vi "main.vi"() -> ()   [LabVIEW 2023] (continued)
FF\tFF\tFF\tFF\tFF\tFF\r\n      2747  1FFFFFFF   00000004    8        00\t00\tFF\tFF\tFF\tFF\tFF\tFF\r\n      2746  18F121F0   00000004    8        09\t19\t00\t00\tFF\tFF\tB0\t01\r\n      2745  18F106A7   00000004    8        00\tF7\tFF\tFF\tFF\tFF\tFF\tA7\r\n      2745  0CF104A7   00000004    8        F0\t60\t22\tFC\tFF\tFF\tFF\t53\r\n      2744  0CF103A7   00000004    8        17\t1F\t08\t60\tB1\t1F\t08\t53\r\n      2783  0CF101A7   00000004    8        68\t00\t97\tCC\t00\t16\t39\tA5\r\n      2782  1FFFFFFF   00000004    8        00\t00\tFF\tFF\tFF\tFF\tFF\tFF\r\n      2772  1FFFFFFF   00000004    8        00\t00\tFF\tFF\tFF\tFF\tFF\tFF\r\n      2763  0CF102A7   00000004    8        30\t75\tE0\t2E\t80\tFF\tFF\tFD\r\n      2763  0CF101A7   00000004    8        68\t00\t97\tCC\t00\t16\t39\tA4\r\n      2762  1FFFFFFF   00000004    8        00\t00\tFF\tFF\tFF\tFF\tFF\tFF\r\n      2752  1FFFFFFF   00000004    8        00\t00\tFF\tFF\tFF\tFF\tFF\tFF\r\n      2747  1FFFFFFF   00000004    8        00\t00\tFF\tFF\tFF\tFF\tFF\tFF\r\n      2746  18F121F0   00000004    8        09\t19\t00\t00\tFF\tFF\tB0\t01\r\n      2745  18F106A7   00000004    8        00\tF7\tFF\tFF\tFF\tFF\tFF\tA7\r\n      2745  0CF104A7   00000004    8        F0\t60\t22\tFC\tFF\tFF\tFF\t53\r\n      2783  0CF102A7   00000004    8        30\t75\tE0\t2E\t80\tFF\tFF\tFD\r\n      2783  0CF101A7   00000004    8        68\t00\t97\tCC\t00\t16\t39\tA5\r\n      2782  1FFFFFFF   00000004    8        00\t00\tFF\tFF\tFF\tFF\tFF\tFF\r\n      2772  1FFFFFFF   00000004    8        00\t00\tFF\tFF\tFF\tFF\tFF\tFF\r\n      2763  0CF102A7   00000004    8        30\t75\tE0\t2E\t80\tFF\tFF\tFD\r\n      2763  0CF101A7   00000004    8        68\t00\t97\tCC\t00\t16\t39\tA4\r\n      2762  1FFFFFFF   00000004    8        00\t00\tFF\tFF\tFF\tFF\tFF\tFF\r\n      2752  1FFFFFFF   00000004    8        00\t00\tFF\tFF\tFF\tFF\tFF\tFF\r\n      2747  1FFFFFFF   00000004    8        00\t00\tFF\tFF\tFF\tFF\tFF\tFF\r\n      2746  18F121F0   00000004    8        09\t19\t00\t00\tFF\tFF\tB0\t01\r\n      2745  18F106A7   00000004    8        00\tF7\tFF\tFF\tFF\tFF\tFF\tA7\r\n      2792  1FFFFFFF   00000004    8        00\t00\tFF\tFF\tFF\tFF\tFF\tFF\r\n      2783  0CF102A7   00000004    8        30\t75\tE0\t2E\t80\tFF\tFF\tFD\r\n      2783  0CF101A7   00000004    8        68\t00\t97\tCC\t00\t16\t39\tA5\r\n      2782  1FFFFFFF   00000004    8        00\t00\tFF\tFF\tFF\tFF\tFF\tFF\r\n      2772  1FFFFFFF   00000004    8        00\t00\tFF\tFF\tFF\tFF\tFF\tFF\r\n      2763  0CF102A7   00000004    8        30\t75\tE0\t2E\t80\tFF\tFF\tFD\r\n      2763  0CF101A7   00000004    8        68\t00\t97\tCC\t00\t16\t39\tA4\r\n      2762  1FFFFFFF   00000004    8        00\t00\tFF\tFF\tFF\tFF\tFF\tFF\r\n      2752  1FFFFFFF   00000004    8        00\t00\tFF\tFF\tFF\tFF\tFF\tFF\r\n      2747  1FFFFFFF   00000004    8        00\t00\tFF\tFF\tFF\tFF\tFF\tFF\r\n      2746  18F121F0   00000004    8        09\t19\t00\t00\tFF\tFF\tB0\t01\r\n      2793  18F106A7   00000004    8        00\tF7\tFF\tFF\tFF\tFF\tFF\tA8\r\n      2792  1FFFFFFF   00000004    8        00\t00\tFF\tFF\tFF\tFF\tFF\tFF\r\n      2783  0CF102A7   00000004    8        30\t75\tE0\t2E\t80\tFF\tFF\tFD\r\n      2783  0CF101A7   00000004    8        68\t00\t97\tCC\t00\t16\t39\tA5\r\n      2782  1FFFFFFF   00000004    8        00\t00\tFF\tFF\tFF\tFF\tFF\tFF\r\n      2772  1FFFFFFF   00000004    8        00\t00\tFF\tFF\tFF\tFF\tFF\tFF\r\n      2763  0CF102A7   00000004    8        30\t75\tE0\t2E\t80\tFF\tFF\tFD\r\n      2763  0CF101A7   00000004    8        68\t00\t97\tCC\t00\t16\t39\tA4\r\n      2762  1FFFFFFF   00000004    8        00\t00\tFF\tFF\tFF\tFF\tFF\tFF\r\n      2752  1FFFFFFF   00000004    8        00\t00\tFF\tFF\tFF\tFF\tFF\tFF\r\n      2747  1FFFFFFF   00000004    8        00\t00\tFF\tFF\tFF\tFF\tFF\tFF\r\n      2802  1FFFFFFF   00000004    8        00\t00\tFF\tFF\tFF\tFF\tFF\tFF\r\n      2793  18F106A7   00000004    8        00\tF7\tFF\tFF\tFF\tFF\tFF\tA8\r\n      2792  1FFFFFFF   00000004    8        00\t00\tFF\tFF\tFF\tFF\tFF\tFF\r\n      2783  0CF102A7   00000004    8        30\t75\tE0\t2E\t80\tFF\tFF\tFD\r\n      2783  0CF101A7   00000004    8        68\t00\t97\tCC\t00\t16\t39\tA5\r\n      2782  1FFFFFFF   00000004    8        00\t00\tFF\tFF\tFF\tFF\tFF\tFF\r\n      2772  1FFFFFFF   00000004    8        00\t00\tFF\tFF\tFF\tFF\tFF\tFF\r\n      2763  0CF102A7   00000004    8        30\t75\tE0\t2E\t80\tFF\tFF\tFD\r\n      2763  0CF101A7   00000004    8        68\t00\t97\tCC\t00\t16\t39\tA4\r\n      2762  1FFFFFFF   00000004    8        00\t00\tFF\tFF\tFF\tFF\tFF\tFF\r\n      2752  1FFFFFFF   00000004    8        00\t00\tFF\tFF\tFF\tFF\tFF\tFF\r\n      2803  0CF101A7   00000004    8        68\t00\t97\tCC\t00\t16\t39\tA6\r\n      2802  1FFFFFFF   00000004    8        00\t00\tFF\tFF\tFF\tFF\tFF\tFF\r\n      2793  18F106A7   00000004    8        00\tF7\tFF\tFF\tFF\tFF\tFF\tA8\r\n      2792  1FFFFFFF   00000004    8        00\t00\tFF\tFF\tFF\tFF\tFF\tFF\r\n      2783  0CF102A7   00000004    8        30\t75\tE0\t2E\t80\tFF\tFF\tFD\r\n      2783  0CF101A7   00000004    8        68\t00\t97\tCC\t00\t16\t39\tA5\r\n      2782  1FFFFFFF   00000004    8        00\t00\tFF\tFF\tFF\tFF\tFF\tFF\r\n      2772  1FFFFFFF   00000004    8        00\t00\tFF\tFF\tFF\tFF\tFF\tFF\r\n      2763  0CF102A7   00000004    8        30\t75\tE0\t2E\t80\tFF\tFF\tFD\r\n      2763  0CF101A7   00000004    8        68\t00\t97\tCC\t00\t16\t39\tA4\r\n      2762  1FFFFFFF   00000004    8        00\t00\tFF\tFF\tFF\tFF\tFF\tFF\r\n      2803  0CF102A7   00000004    8        30\t75\tE0\t2E\t80\tFF\tFF\tFD\r\n      2803  0CF101A7   00000004    8        68\t00\t97\tCC\t00\t16\t39\tA6\r\n      2802  1FFFFFFF   00000004    8        00\t00\tFF\tFF\tFF\tFF\tFF\tFF\r\n      2793  18F106A7   00000004    8        00\tF7\tFF\tFF\tFF\tFF\tFF\tA8\r\n      2792  1FFFFFFF   00000004    8        00\t00\tFF\tFF\tFF\tFF\tFF\tFF\r\n      2783  0CF102A7   00000004    8        30\t75\tE0\t2E\t80\tFF\tFF\tFD\r\n      2783  0CF101A7   00000004    8        68\t00\t97\tCC\t00\t16\t39\tA5\r\n      2782  1FFFFFFF   00000004    8        00\t00\tFF\tFF\tFF\tFF\tFF\tFF\r\n      2772  1FFFFFFF   00000004    8        00\t00\tFF\tFF\tFF\tFF\tFF\tFF\r\n      2763  0CF102A7   00000004    8        30\t75\tE0\t2E\t80\tFF\tFF\tFD\r\n      2763  0CF101A7   00000004    8        68\t00\t97\tCC\t00\t16\t39\tA4\r\n      2812  1FFFFFFF   00000004    8        00\t00\tFF\tFF\tFF\tFF\tFF\tFF\r\n      2803  0CF102A7   00000004    8        30\t75\tE0\t2E\t80\tFF\tFF\tFD\r\n      2803  0CF101A7   00000004    8        68\t00\t97\tCC\t00\t16\t39\tA6\r\n      2802  1FFFFFFF   00000004    8        00\t00\tFF\tFF\tFF\tFF\tFF\tFF\r\n      2793  18F106A7   00000004    8        00\tF7\tFF\tFF\tFF\tFF\tFF\tA8\r\n      2792  1FFFFFFF   00000004    8        00\t00\tFF\tFF\tFF\tFF\tFF\tFF\r\n      2783  0CF102A7   00000004    8        30\t75\tE0\t2E\t80\tFF\tFF\tFD\r\n      2783  0CF101A7   00000004    8        68\t00\t97\tCC\t00\t16\t39\tA5\r\n      2782  1FFFFFFF   00000004    8        00\t00\tFF\tFF\tFF\tFF\tFF\tFF\r\n      2772  1FFFFFFF   00000004    8        00\t00\tFF\tFF\tFF\tFF\tFF\tFF\r\n      2763  0CF102A7   00000004    8        30\t75\tE0\t2E\t80\tFF\tFF\tFD\r\n      2822  1FFFFFFF   00000004    8        00\t00\tFF\tFF\tFF\tFF\tFF\tFF\r\n      2812  1FFFFFFF   00000004    8        00\t00\tFF\tFF\tFF\tFF\tFF\tFF\r\n      2803  0CF102A7   00000004    8        30\t75\tE0\t2E\t80\tFF\tFF\tFD\r\n      2803  0CF101A7   00000004    8        68\t00\t97\tCC\t00\t16\t39\tA6\r\n      2802  1FFFFFFF   00000004    8        00\t00\tFF\tFF\tFF\tFF\tFF\tFF\r\n      2793  18F106A7   00000004    8        00\tF7\tFF\tFF\tFF\tFF\tFF\tA8\r\n      2792  1FFFFFFF   00000004    8        00\t00\tFF\tFF\tFF\tFF\tFF\tFF\r\n      2783  0CF102A7   00000004    8        30\t75\tE0\t2E\t80\tFF\tFF\tFD\r\n      2783  0CF101A7   00000004    8        68\t00\t97\tCC\t00\t16\t39\tA5\r\n      2782  1FFFFFFF   00000004    8        00\t00\tFF\tFF\tFF\tFF\tFF\tFF\r\n      2772  1FFFFFFF   00000004    8        00\t00\tFF\tFF\tFF\tFF\tFF\tFF\r\n      2823  0CF101A7   00000004    8        68\t00\t97\tCC\t00\t16\t39\tA7\r\n      2822  1FFFFFFF   00000004    8        00\t00\tFF\tFF\tFF\tFF\tFF\tFF\r\n      2812  1FFFFFFF   00000004    8        00\t00\tFF\tFF\tFF\tFF\tFF\tFF\r\n      2803  0CF102A7   00000004    8        30\t75\tE0\t2E\t80\tFF\tFF\tFD\r\n      2803  0CF101A7   00000004    8        68\t00\t97\tCC\t00\t16\t39\tA6\r\n      2802  1FFFFFFF   00000004    8        00\t00\tFF\tFF\tFF\tFF\tFF\tFF\r\n      2793  18F106A7   00000004    8        00\tF7\tFF\tFF\tFF\tFF\tFF\tA8\r\n      2792  1FFFFFFF   00000004    8        00\t00\tFF\tFF\tFF\tFF\tFF\tFF\r\n      2783  0CF102A7   00000004    8        30\t75\tE0\t2E\t80\tFF\tFF\tFD\r\n      2783  0CF101A7   00000004    8        68\t00\t97\tCC\t00\t16\t39\tA5\r\n      2782  1FFFFFFF   00000004    8        00\t00\tFF\tFF\tFF\tFF\tFF\tFF\r\n      2823  0CF102A7   00000004    8        30\t75\tE0\t2E\t80\tFF\tFF\tFD\r\n      2823  0CF101A7   00000004    8        68\t00\t97\tCC\t00\t16\t39\tA7\r\n      2822  1FFFFFFF   00000004    8        00\t00\tFF\tFF\tFF\tFF\tFF\tFF\r\n      2812  1FFFFFFF   00000004    8        00\t00\tFF\tFF\tFF\tFF\tFF\tFF\r\n      2803  0CF102A7   00000004    8        30\t75\tE0\t2E\t80\tFF\tFF\tFD\r\n      2803  0CF101A7   00000004    8        68\t00\t97\tCC\t00\t16\t39\tA6\r\n      2802  1FFFFFFF   00000004    8        00\t00\tFF\tFF\tFF\tFF\tFF\tFF\r\n      2793  18F106A7   00000004    8        00\tF7\tFF\tFF\tFF\tFF\tFF\tA8\r\n      2792  1FFFFFFF   00000004    8        00\t00\tFF\tFF\tFF\tFF\tFF\tFF\r\n      2783  0CF102A7   00000004    8        30\t75\tE0\t2E\t80\tFF\tFF\tFD\r\n      2783  0CF101A7   00000004    8        68\t00\t97\tCC\t00\t16\t39\tA5\r\n      2832  1FFFFFFF   00000004    8        00\t00\tFF\tFF\tFF\tFF\tFF\tFF\r\n      2823  0CF102A7   00000004    8        30\t75\tE0\t2E\t80\tFF\tFF\tFD\r\n      2823  0CF101A7   00000004    8        68\t00\t97\tCC\t00\t16\t39\tA7\r\n      2822  1FFFFFFF   00000004    8        00\t00\tFF\tFF\tFF\tFF\tFF\tFF\r\n      2812  1FFFFFFF   00000004    8        00\t00\tFF\tFF\tFF\tFF\tFF\tFF\r\n      2803  0CF102A7   00000004    8        30\t75\tE0\t2E\t80\tFF\tFF\tFD\r\n      2803  0CF101A7   00000004    8        68\t00\t97\tCC\t00\t16\t39\tA6\r\n      2802  1FFFFFFF   00000004    8        00\t00\tFF\tFF\tFF\tFF\tFF\tFF\r\n      2793  18F106A7   00000004    8        00\tF7\tFF\tFF\tFF\tFF\tFF\tA8\r\n      2792  1FFFFFFF   00000004    8        00\t00\tFF\tFF\tFF\tFF\tFF\tFF\r\n      2783  0CF102A7   00000004    8        30\t75\tE0\t2E\t80\tFF\tFF\tFD\r\n      2841  18F11FF0   00000004    8        FF\t3F\t90\t68\t88\t1B\t10\t4C\r\n      2832  1FFFFFFF   00000004    8        00\t00\tFF\tFF\tFF\tFF\tFF\tFF\r\n      2823  0CF102A7   00000004    8        30\t75\tE0\t2E\t80\tFF\tFF\tFD\r\n      2823  0CF101A7   00000004    8        68\t00\t97\tCC\t00\t16\t39\tA7\r\n      2822  1FFFFFFF   00000004    8        00\t00\tFF\tFF\tFF\tFF\tFF\tFF\r\n      2812  1FFFFFFF   00000004    8        00\t00\tFF\tFF\tFF\tFF\tFF\tFF\r\n      2803  0CF102A7   00000004    8        30\t75\tE0\t2E\t80\tFF\tFF\tFD\r\n      2803  0CF101A7   00000004    8        68\t00\t97\tCC\t00\t16\t39\tA6\r\n      2802  1FFFFFFF   00000004    8        00\t00\tFF\tFF\tFF\tFF\tFF\tFF\r\n      2793  18F106A7   00000004    8        00\tF7\tFF\tFF\tFF\tFF\tFF\tA8\r\n      2792  1FFFFFFF   00000004    8        00\t00\tFF\tFF\tFF\tFF\tFF\tFF\r\n      2842  18F120F0   00000004    8        2B\t75\t60\tB1\tB0\t01\tFF\tFF\r\n      2841  18F11FF0   00000004    8        FF\t3F\t90\t68\t88\t1B\t10\t4C\r\n      2832  1FFFFFFF   00000004    8        00\t00\tFF\tFF\tFF\tFF\tFF\tFF\r\n      2823  0CF102A7   00000004    8        30\t75\tE0\t2E\t80\tFF\tFF\tFD\r\n      2823  0CF101A7   00000004    8        68\t00\t97\tCC\t00\t16\t39\tA7\r\n      2822  1FFFFFFF   00000004    8        00\t00\tFF\tFF\tFF\tFF\tFF\tFF\r\n      2812  1FFFFFFF   00000004    8        00\t00\tFF\tFF\tFF\tFF\tFF\tFF\r\n      2803  0CF102A7   00000004    8        30\t75\tE0\t2E\t80\tFF\tFF\tFD\r\n      2803  0CF101A7   00000004    8        68\t00\t97\tCC\t00\t16\t39\tA6\r\n      2802  1FFFFFFF   00000004    8        00\t00\tFF\tFF\tFF\tFF\tFF\tFF\r\n      2793  18F106A7   00000004    8        00\tF7\tFF\tFF\tFF\tFF\tFF\tA8\r\n      2843  0CF101A7   00000004    8        68\t00\t97\tCC\t00\t16\t39\tA8\r\n      2842  18F120F0   00000004    8        2B\t75\t60\tB1\tB0\t01\tFF\tFF\r\n      2841  18F11FF0   00000004    8        FF\t3F\t90\t68\t88\t1B\t10\t4C\r\n      2832  1FFFFFFF   00000004    8        00\t00\tFF\tFF\tFF\tFF\tFF\tFF\r\n      2823  0CF102A7   00000004    8        30\t75\tE0\t2E\t80\tFF\tFF\tFD\r\n      2823  0CF101A7   00000004    8        68\t00\t97\tCC\t00\t16\t39\tA7\r\n      2822  1FFFFFFF   00000004    8        00\t00\tFF\tFF\tFF\tFF\tFF\tFF\r\n      2812  1FFFFFFF   00000004    8        00\t00\tFF\tFF\tFF\tFF\tFF\tFF\r\n      2803  0CF102A7   00000004    8        30\t75\tE0\t2E\t80\tFF\tFF\tFD\r\n      2803  0CF101A7   00000004    8        68\t00\t97\tCC\t00\t16\t39\tA6\r\n      2802  1FFFFFFF   00000004    8        00\t00\tFF\tFF\tFF\tFF\tFF\tFF\r\n      2843  0C3C4D4A   00000004    8        BE\tFF\tFF\t7F\t18\tFF\tFF\t54\r\n      2843  0CF101A7   00000004    8        68\t00\t97\tCC\t00\t16\t39\tA8\r\n      2842  18F120F0   00000004    8        2B\t75\t60\tB1\tB0\t01\tFF\tFF\r\n      2841  18F11FF0   00000004    8        FF\t3F\t90\t68\t88\t1B\t10\t4C\r\n      2832  1FFFFFFF   00000004    8        00\t00\tFF\tFF\tFF\tFF\tFF\tFF\r\n      2823  0CF102A7   00000004    8        30\t75\tE0\t2E\t80\tFF\tFF\tFD\r\n      2823  0CF101A7   00000004    8        68\t00\t97\tCC\t00\t16\t39\tA7\r\n      2822  1FFFFFFF   00000004    8        00\t00\tFF\tFF\tFF\tFF\tFF\tFF\r\n      2812  1FFFFFFF   00000004    8        00\t00\tFF\tFF\tFF\tFF\tFF\tFF\r\n      2803  0CF102A7   00000004    8        30\t75\tE0\t2E\t80\tFF\tFF\tFD\r\n      2803  0CF101A7   00000004    8        68\t00\t97\tCC\t00\t16\t39\tA6\r\n      2844  0CF102A7   00000004    8        30\t75\tE0\t2E\t80\tFF\tFF\tFD\r\n      2843  0C3C4D4A   00000004    8        BE\tFF\tFF\t7F\t18\tFF\tFF\t54\r\n      2843  0CF101A7   00000004    8        68\t00\t97\tCC\t00\t16\t39\tA8\r\n      2842  18F120F0   00000004    8        2B\t75\t60\tB1\tB0\t01\tFF\tFF\r\n      2841  18F11FF0   00000004    8        FF\t3F\t90\t68\t88\t1B\t10\t4C\r\n      2832  1FFFFFFF   00000004    8        00\t00\tFF\tFF\tFF\tFF\tFF\tFF\r\n      2823  0CF102A7   00000004    8        30\t75\tE0\t2E\t80\tFF\tFF\tFD\r\n      2823  0CF101A7   00000004    8        68\t00\t97\tCC\t00\t16\t39\tA7\r\n      2822  1FFFFFFF   00000004    8        00\t00\tFF\tFF\tFF\tFF\tFF\tFF\r\n      2812  1FFFFFFF   00000004    8        00\t00\tFF\tFF\tFF\tFF\tFF\tFF\r\n      2803  0CF102A7   00000004    8        30\t75\tE0\t2E\t80\tFF\tFF\tFD\r\n      2844  0CF103A7   00000004    8        17\t1F\t08\t60\tB1\t1F\t08\t54\r\n      2844  0CF102A7   00000004    8        30\t75\tE0\t2E\t80\tFF\tFF\tFD\r\n      2843  0C3C4D4A   00000004    8        BE\tFF\tFF\t7F\t18\tFF\tFF\t54\r\n      2843  0CF101A7   00000004    8        68\t00\t97\tCC\t00\t16\t39\tA8\r\n      2842  18F120F0   00000004    8        2B\t75\t60\tB1\tB0\t01\tFF\tFF\r\n      2841  18F11FF0   00000004    8        FF\t3F\t90\t68\t88\t1B\t10\t4C\r\n      2832  1FFFFFFF   00000004    8        00\t00\tFF\tFF\tFF\tFF\tFF\tFF\r\n      2823  0CF102A7   00000004    8        30\t75\tE0\t2E\t80\tFF\tFF\tFD\r\n      2823  0CF101A7   00000004    8        68\t00\t97\tCC\t00\t16\t39\tA7\r\n      2822  1FFFFFFF   00000004    8        00\t00\tFF\tFF\tFF\tFF\tFF\tFF\r\n      2812  1FFFFFFF   00000004    8        00\t00\tFF\tFF\tFF\tFF\tFF\tFF\r\n      2845  0CF104A7   00000004    8        F0\t60\t22\tFC\tFF\tFF\tFF\t54\r\n      2844  0CF103A7   00000004    8        17\t1F\t08\t60\tB1\t1F\t08\t54\r\n      2844  0CF102A7   00000004    8        30\t75\tE0\t2E\t80\tFF\tFF\tFD\r\n      2843  0C3C4D4A   00000004    8        BE\tFF\tFF\t7F\t18\tFF\tFF\t54\r\n      2843  0CF101A7   00000004    8        68\t00\t97\tCC\t00\t16\t39\tA8\r\n      2842  18F120F0   00000004    8        2B\t75\t60\tB1\tB0\t01\tFF\tFF\r\n      2841  18F11FF0   00000004    8        FF\t3F\t90\t68\t88\t1B\t10\t4C\r\n      2832  1FFFFFFF   00000004    8        00\t00\tFF\tFF\tFF\tFF\tFF\tFF\r\n      2823  0CF102A7   00000004    8        30\t75\tE0\t2E\t80\tFF\tFF\tFD\r\n      2823  0CF101A7   00000004    8        68\t00\t97\tCC\t00\t16\t39\tA7\r\n      2822  1FFFFFFF   00000004    8        00\t00\tFF\tFF\tFF\tFF\tFF\tFF\r\n      2845  18F106A7   00000004    8        00\tF7\tFF\tFF\tFF\tFF\tFF\tA9\r\n      2845  0CF104A7   00000004    8        F0\t60\t22\tFC\tFF\tFF\tFF\t54\r\n      2844  0CF103A7   00000004    8        17\t1F\t08\t60\tB1\t1F\t08\t54\r\n      2844  0CF102A7   00000004    8        30\t75\tE0\t2E\t80\tFF\tFF\tFD\r\n      2843  0C3C4D4A   00000004    8        BE\tFF\tFF\t7F\t18\tFF\tFF\t54\r\n      2843  0CF101A7   00000004    8        68\t00\t97\tCC\t00\t16\t39\tA8\r\n      2842  18F120F0   00000004    8        2B\t75\t60\tB1\tB0\t01\tFF\tFF\r\n      2841  18F11FF0   00000004    8        FF\t3F\t90\t68\t88\t1B\t10\t4C\r\n      2832  1FFFFFFF   00000004    8        00\t00\tFF\tFF\tFF\tFF\tFF\tFF\r\n      2823  0CF102A7   00000004    8        30\t75\tE0\t2E\t80\tFF\tFF\tFD\r\n      2823  0CF101A7   00000004    8        68\t00\t97\tCC\t00\t16\t39\tA7\r\n      2846  18F121F0   00000004    8        09\t19\t00\t00\tFF\tFF\tB0\t01\r\n      2845  18F106A7   00000004    8        00\tF7\tFF\tFF\tFF\tFF\tFF\tA9\r\n      2845  0CF104A7   00000004    8        F0\t60\t22\tFC\tFF\tFF\tFF\t54\r\n      2844  0CF103A7   00000004    8        17\t1F\t08\t60\tB1\t1F\t08\t54\r\n      2844  0CF102A7   00000004    8        30\t75\tE0\t2E\t80\tFF\tFF\tFD\r\n      2843  0C3C4D4A   00000004    8        BE\tFF\tFF\t7F\t18\tFF\tFF\t54\r\n      2843  0CF101A7   00000004    8        68\t00\t97\tCC\t00\t16\t39\tA8\r\n      2842  18F120F0   00000004    8        2B\t75\t60\tB1\tB0\t01\tFF\tFF\r\n      2841  18F11FF0   00000004    8        FF\t3F\t90\t68\t88\t1B\t10\t4C\r\n      2832  1FFFFFFF   00000004    8        00\t00\tFF\tFF\tFF\tFF\tFF\tFF\r\n      2823  0CF102A7   00000004    8        30\t75\tE0\t2E\t80\tFF\tFF\tFD\r\n      2847  1FFFFFFF   00000004    8        00\t00\tFF\tFF\tFF\tFF\tFF\tFF\r\n      2846  18F121F0   00000004    8        09\t19\t00\t00\tFF\tFF\tB0\t01\r\n      2845  18F106A7   00000004    8        00\tF7\tFF\tFF\tFF\tFF\tFF\tA9\r\n      2845  0CF104A7   00000004    8        F0\t60\t22\tFC\tFF\tFF\tFF\t54\r\n      2844  0CF103A7   00000004    8        17\t1F\t08\t60\tB1\t1F\t08\t54\r\n      2844  0CF102A7   00000004    8        30\t75\tE0\t2E\t80\tFF\tFF\tFD\r\n      2843  0C3C4D4A   00000004    8        BE\tFF\tFF\t7F\t18\tFF\tFF\t54\r\n      2843  0CF101A7   00000004    8        68\t00\t97\tCC\t00\t16\t39\tA8\r\n      2842  18F120F0   00000004    8        2B\t75\t60\tB1\tB0\t01\tFF\tFF\r\n      2841  18F11FF0   00000004    8        FF\t3F\t90\t68\t88\t1B\t10\t4C\r\n      2832  1FFFFFFF   00000004    8        00\t00\tFF\tFF\tFF\tFF\tFF\tFF\r\n      2852  1FFFFFFF   00000004    8        00\t20\tFF\tFF\tFF\tFF\tFF\tFF\r\n      2847  1FFFFFFF   00000004    8        00\t00\tFF\tFF\tFF\tFF\tFF\tFF\r\n      2846  18F121F0   00000004    8        09\t19\t00\t00\tFF\tFF\tB0\t01\r\n      2845  18F106A7   00000004    8        00\tF7\tFF\tFF\tFF\tFF\tFF\tA9\r\n      2845  0CF104A7   00000004    8        F0\t60\t22\tFC\tFF\tFF\tFF\t54\r\n      2844  0CF103A7   00000004    8        17\t1F\t08\t60\tB1\t1F\t08\t54\r\n      2844  0CF102A7   00000004    8        30\t75\tE0\t2E\t80\tFF\tFF\tFD\r\n      2843  0C3C4D4A   00000004    8        BE\tFF\tFF\t7F\t18\tFF\tFF\t54\r\n      2843  0CF101A7   00000004    8        68\t00\t97\tCC\t00\t16\t39\tA8\r\n      2842  18F120F0   00000004    8        2B\t75\t60\tB1\tB0\t01\tFF\tFF\r\n      2841  18F11FF0   00000004    8        FF\t3F\t90\t68\t88\t1B\t10\t4C\r\n      2862  1FFFFFFF   00000004    8        00\t20\tFF\tFF\tFF\tFF\tFF\tFF\r\n      2852  1FFFFFFF   00000004    8        00\t20\tFF\tFF\tFF\tFF\tFF\tFF\r\n      2847  1FFFFFFF   00000004    8        00\t00\tFF\tFF\tFF\tFF\tFF\tFF\r\n      2846  18F121F0   00000004    8        09\t19\t00\t00\tFF\tFF\tB0\t01\r\n      2845  18F106A7   00000004    8        00\tF7\tFF\tFF\tFF\tFF\tFF\tA9\r\n      2845  0CF104A7   00000004    8        F0\t60\t22\tFC\tFF\tFF\tFF\t54\r\n      2844  0CF103A7   00000004    8        17\t1F\t08\t60\tB1\t1F\t08\t54\r\n      2844  0CF102A7   00000004    8        30\t75\tE0\t2E\t80\tFF\tFF\tFD\r\n      2843  0C3C4D4A   00000004    8        BE\tFF\tFF\t7F\t18\tFF\tFF\t54\r\n      2843  0CF101A7   00000004    8        68\t00\t97\tCC\t00\t16\t39\tA8\r\n      2842  18F120F0   00000004    8        2B\t75\t60\tB1\tB0\t01\tFF\tFF\r\n      2863  0CF101A7   00000004    8        68\t00\t97\tCC\t00\t16\t39\tA9\r\n      2862  1FFFFFFF   00000004    8        00\t20\tFF\tFF\tFF\tFF\tFF\tFF\r\n      2852  1FFFFFFF   00000004    8        00\t20\tFF\tFF\tFF\tFF\tFF\tFF\r\n      2847  1FFFFFFF   00000004    8        00\t00\tFF\tFF\tFF\tFF\tFF\tFF\r\n      2846  18F121F0   00000004    8        09\t19\t00\t00\tFF\tFF\tB0\t01\r\n      2845  18F106A7   00000004    8        00\tF7\tFF\tFF\tFF\tFF\tFF\tA9\r\n      2845  0CF104A7   00000004    8        F0\t60\t22\tFC\tFF\tFF\tFF\t54\r\n      2844  0CF103A7   00000004    8        17\t1F\t08\t60\tB1\t1F\t08\t54\r\n      2844  0CF102A7   00000004    8        30\t75\tE0\t2E\t80\tFF\tFF\tFD\r\n      2843  0C3C4D4A   00000004    8        BE\tFF\tFF\t7F\t18\tFF\tFF\t54\r\n      2843  0CF101A7   00000004    8        68\t00\t97\tCC\t00\t16\t39\tA8\r\n      2863  0CF102A7   00000004    8        30\t75\tE0\t2E\t80\tFF\tFF\tFD\r\n      2863  0CF101A7   00000004    8        68\t00\t97\tCC\t00\t16\t39\tA9\r\n      2862  1FFFFFFF   00000004    8        00\t20\tFF\tFF\tFF\tFF\tFF\tFF\r\n      2852  1FFFFFFF   00000004    8        00\t20\tFF\tFF\tFF\tFF\tFF\tFF\r\n      2847  1FFFFFFF   00000004    8        00\t00\tFF\tFF\tFF\tFF\tFF\tFF\r\n      2846  18F121F0   00000004    8        09\t19\t00\t00\tFF\tFF\tB0\t01\r\n      2845  18F106A7   00000004    8        00\tF7\tFF\tFF\tFF\tFF\tFF\tA9\r\n      2845  0CF104A7   00000004    8        F0\t60\t22\tFC\tFF\tFF\tFF\t54\r\n      2844  0CF103A7   00000004    8        17\t1F\t08\t60\tB1\t1F\t08\t54\r\n      2844  0CF102A7   00000004    8        30\t75\tE0\t2E\t80\tFF\tFF\tFD\r\n      2843  0C3C4D4A   00000004    8        BE\tFF\tFF\t7F\t18\tFF\tFF\t54\r\n      2872  1FFFFFFF   00000004    8        00\t00\tFF\tFF\tFF\tFF\tFF\tFF\r\n      2863  0CF102A7   00000004    8        30\t75\tE0\t2E\t80\tFF\tFF\tFD\r\n      2863  0CF101A7   00000004    8        68\t00\t97\tCC\t00\t16\t39\tA9\r\n      2862  1FFFFFFF   00000004    8        00\t20\tFF\tFF\tFF\tFF\tFF\tFF\r\n      2852  1FFFFFFF   00000004    8        00\t20\tFF\tFF\tFF\tFF\tFF\tFF\r\n      2847  1FFFFFFF   00000004    8        00\t00\tFF\tFF\tFF\tFF\tFF\tFF\r\n      2846  18F121F0   00000004    8        09\t19\t00\t00\tFF\tFF\tB0\t01\r\n      2845  18F106A7   00000004    8        00\tF7\tFF\tFF\tFF\tFF\tFF\tA9\r\n      2845  0CF104A7   00000004    8        F0\t60\t22\tFC\tFF\tFF\tFF\t54\r\n      2844  0CF103A7   00000004    8        17\t1F\t08\t60\tB1\t1F\t08\t54\r\n      2844  0CF102A7   00000004    8        30\t75\tE0\t2E\t80\tFF\tFF\tFD\r\n      2882  1FFFFFFF   00000004    8        00\t00\tFF\tFF\tFF\tFF\tFF\tFF\r\n      2872  1FFFFFFF   00000004    8        00\t00\tFF\tFF\tFF\tFF\tFF\tFF\r\n      2863  0CF102A7   00000004    8        30\t75\tE0\t2E\t80\tFF\tFF\tFD\r\n      2863  0CF101A7   00000004    8        68\t00\t97\tCC\t00\t16\t39\tA9\r\n      2862  1FFFFFFF   00000004    8        00\t20\tFF\tFF\tFF\tFF\tFF\tFF\r\n      2852  1FFFFFFF   00000004    8        00\t20\tFF\tFF\tFF\tFF\tFF\tFF\r\n      2847  1FFFFFFF   00000004    8        00\t00\tFF\tFF\tFF\tFF\tFF\tFF\r\n      2846  18F121F0   00000004    8        09\t19\t00\t00\tFF\tFF\tB0\t01\r\n      2845  18F106A7   00000004    8        00\tF7\tFF\tFF\tFF\tFF\tFF\tA9\r\n      2845  0CF104A7   00000004    8        F0\t60\t22\tFC\tFF\tFF\tFF\t54\r\n      2844  0CF103A7   00000004    8        17\t1F\t08\t60\tB1\t1F\t08\t54\r\n      2883  0CF101A7   00000004    8        68\t00\t97\tCC\t00\t16\t39\tAA\r\n      2882  1FFFFFFF   00000004    8        00\t00\tFF\tFF\tFF\tFF\tFF\tFF\r\n      2872  1FFFFFFF   00000004    8        00\t00\tFF\tFF\tFF\tFF\tFF\tFF\r\n      2863  0CF102A7   00000004    8        30\t75\tE0\t2E\t80\tFF\tFF\tFD\r\n      2863  0CF101A7   00000004    8        68\t00\t97\tCC\t00\t16\t39\tA9\r\n      2862  1FFFFFFF   00000004    8        00\t20\tFF\tFF\tFF\tFF\tFF\tFF\r\n      2852  1FFFFFFF   00000004    8        00\t20\tFF\tFF\tFF\tFF\tFF\tFF\r\n      2847  1FFFFFFF   00000004    8        00\t00\tFF\tFF\tFF\tFF\tFF\tFF\r\n      2846  18F121F0   00000004    8        09\t19\t00\t00\tFF\tFF\tB0\t01\r\n      2845  18F106A7   00000004    8        00\tF7\tFF\tFF\tFF\tFF\tFF\tA9\r\n      2845  0CF104A7   00000004    8        F0\t60\t22\tFC\tFF\tFF\tFF\t54\r\n      2883  0CF102A7   00000004    8        30\t75\tE0\t2E\t80\tFF\tFF\tFD\r\n      2883  0CF101A7   00000004    8        68\t00\t97\tCC\t00\t16\t39\tAA\r\n      2882  1FFFFFFF   00000004    8        00\t00\tFF\tFF\tFF\tFF\tFF\tFF\r\n      2872  1FFFFFFF   00000004    8        00\t00\tFF\tFF\tFF\tFF\tFF\tFF\r\n      2863  0CF102A7   00000004    8        30\t75\tE0\t2E\t80\tFF\tFF\tFD\r\n      2863  0CF101A7   00000004    8        68\t00\t97\tCC\t00\t16\t39\tA9\r\n      2862  1FFFFFFF   00000004    8        00\t20\tFF\tFF\tFF\tFF\tFF\tFF\r\n      2852  1FFFFFFF   00000004    8        00\t20\tFF\tFF\tFF\tFF\tFF\tFF\r\n      2847  1FFFFFFF   00000004    8        00\t00\tFF\tFF\tFF\tFF\tFF\tFF\r\n      2846  18F121F0   00000004    8        09\t19\t00\t00\tFF\tFF\tB0\t01\r\n      2845  18F106A7   00000004    8        00\tF7\tFF\tFF\tFF\tFF\tFF\tA9\r\n      2892  1FFFFFFF   00000004    8        00\t20\tFF\tFF\tFF\tFF\tFF\tFF\r\n      2883  0CF102A7   00000004    8        30\t75\tE0\t2E\t80\tFF\tFF\tFD\r\n      2883  0CF101A7   00000004    8        68\t00\t97\tCC\t00\t16\t39\tAA\r\n      2882  1FFFFFFF   00000004    8        00\t00\tFF\tFF\tFF\tFF\tFF\tFF\r\n      2872  1FFFFFFF   00000004    8        00\t00\tFF\tFF\tFF\tFF\tFF\tFF\r\n      2863  0CF102A7   00000004    8        30\t75\tE0\t2E\t80\tFF\tFF\tFD\r\n      2863  0CF101A7   00000004    8        68\t00\t97\tCC\t00\t16\t39\tA9\r\n      2862  1FFFFFFF   00000004    8        00\t20\tFF\tFF\tFF\tFF\tFF\tFF\r\n      2852  1FFFFFFF   00000004    8        00\t20\tFF\tFF\tFF\tFF\tFF\tFF\r\n      2847  1FFFFFFF   00000004    8        00\t00\tFF\tFF\tFF\tFF\tFF\tFF\r\n      2846  18F121F0   00000004    8        09\t19\t00\t00\tFF\tFF\tB0\t01\r\n      2893  18F106A7   00000004    8        00\tF7\tFF\tFF\tFF\tFF\tFF\tAA\r\n      2892  1FFFFFFF   00000004    8        00\t20\tFF\tFF\tFF\tFF\tFF\tFF\r\n      2883  0CF102A7   00000004    8        30\t75\tE0\t2E\t80\tFF\tFF\tFD\r\n      2883  0CF101A7   00000004    8        68\t00\t97\tCC\t00\t16\t39\tAA\r\n      2882  1FFFFFFF   00000004    8        00\t00\tFF\tFF\tFF\tFF\tFF\tFF\r\n      2872  1FFFFFFF   00000004    8        00\t00\tFF\tFF\tFF\tFF\tFF\tFF\r\n      2863  0CF102A7   00000004    8        30\t75\tE0\t2E\t80\tFF\tFF\tFD\r\n      2863  0CF101A7   00000004    8        68\t00\t97\tCC\t00\t16\t39\tA9\r\n      2862  1FFFFFFF   00000004    8        00\t20\tFF\tFF\tFF\tFF\tFF\tFF\r\n      2852  1FFFFFFF   00000004    8        00\t20\tFF\tFF\tFF\tFF\tFF\tFF\r\n      2847  1FFFFFFF   00000004    8        00\t00\tFF\tFF\tFF\tFF\tFF\tFF\r\n      2902  1FFFFFFF   00000004    8        00\t20\tFF\tFF\tFF\tFF\tFF\tFF\r\n      2893  18F106A7   00000004    8        00\tF7\tFF\tFF\tFF\tFF\tFF\tAA\r\n      2892  1FFFFFFF   00000004    8        00\t20\tFF\tFF\tFF\tFF\tFF\tFF\r\n      2883  0CF102A7   00000004    8        30\t75\tE0\t2E\t80\tFF\tFF\tFD\r\n      2883  0CF101A7   00000004    8        68\t00\t97\tCC\t00\t16\t39\tAA\r\n      2882  1FFFFFFF   00000004    8        00\t00\tFF\tFF\tFF\tFF\tFF\tFF\r\n      2872  1FFFFFFF   00000004    8        00\t00\tFF\tFF\tFF\tFF\tFF\tFF\r\n      2863  0CF102A7   00000004    8        30\t75\tE0\t2E\t80\tFF\tFF\tFD\r\n      2863  0CF101A7   00000004    8        68\t00\t97\tCC\t00\t16\t39\tA9\r\n      2862  1FFFFFFF   00000004    8        00\t20\tFF\tFF\tFF\tFF\tFF\tFF\r\n      2852  1FFFFFFF   00000004    8        00\t20\tFF\tFF\tFF\tFF\tFF\tFF\r\n      2903  0CF101A7   00000004    8        68\t00\t97\tCC\t00\t16\t39\tAB\r\n      2902  1FFFFFFF   00000004    8        00\t20\tFF\tFF\tFF\tFF\tFF\tFF\r\n      2893  18F106A7   00000004    8        00\tF7\tFF\tFF\tFF\tFF\tFF\tAA\r\n      2892  1FFFFFFF   00000004    8        00\t20\tFF\tFF\tFF\tFF\tFF\tFF\r\n      2883  0CF102A7   00000004    8        30\t75\tE0\t2E\t80\tFF\tFF\tFD\r\n      2883  0CF101A7   00000004    8        68\t00\t97\tCC\t00\t16\t39\tAA\r\n      2882  1FFFFFFF   00000004    8        00\t00\tFF\tFF\tFF\tFF\tFF\tFF\r\n      2872  1FFFFFFF   00000004    8        00\t00\tFF\tFF\tFF\tFF\tFF\tFF\r\n      2863  0CF102A7   00000004    8        30\t75\tE0\t2E\t80\tFF\tFF\tFD\r\n      2863  0CF101A7   00000004    8        68\t00\t97\tCC\t00\t16\t39\tA9\r\n      2862  1FFFFFFF   00000004    8        00\t20\tFF\tFF\tFF\tFF\tFF\tFF\r\n      2903  0CF102A7   00000004    8        30\t75\tE0\t2E\t80\tFF\tFF\tFD\r\n      2903  0CF101A7   00000004    8        68\t00\t97\tCC\t00\t16\t39\tAB\r\n      2902  1FFFFFFF   00000004    8        00\t20\tFF\tFF\tFF\tFF\tFF\tFF\r\n      2893  18F106A7   00000004    8        00\tF7\tFF\tFF\tFF\tFF\tFF\tAA\r\n      2892  1FFFFFFF   00000004    8        00\t20\tFF\tFF\tFF\tFF\tFF\tFF\r\n      2883  0CF102A7   00000004    8        30\t75\tE0\t2E\t80\tFF\tFF\tFD\r\n      2883  0CF101A7   00000004    8        68\t00\t97\tCC\t00\t16\t39\tAA\r\n      2882  1FFFFFFF   00000004    8        00\t00\tFF\tFF\tFF\tFF\tFF\tFF\r\n      2872  1FFFFFFF   00000004    8        00\t00\tFF\tFF\tFF\tFF\tFF\tFF\r\n      2863  0CF102A7   00000004    8        30\t75\tE0\t2E\t80\tFF\tFF\tFD\r\n      2863  0CF101A7   00000004    8        68\t00\t97\tCC\t00\t16\t39\tA9\r\n      2912  1FFFFFFF   00000004    8        00\t20\tFF\tFF\tFF\tFF\tFF\tFF\r\n      2903  0CF102A7   00000004    8        30\t75\tE0\t2E\t80\tFF\tFF\tFD\r\n      2903  0CF101A7   00000004    8        68\t00\t97\tCC\t00\t16\t39\tAB\r\n      2902  1FFFFFFF   00000004    8        00\t20\tFF\tFF\tFF\tFF\tFF\tFF\r\n      2893  18F106A7   00000004    8        00\tF7\tFF\tFF\tFF\tFF\tFF\tAA\r\n      2892  1FFFFFFF   00000004    8        00\t20\tFF\tFF\tFF\tFF\tFF\tFF\r\n      2883  0CF102A7   00000004    8        30\t75\tE0\t2E\t80\tFF\tFF\tFD\r\n      2883  0CF101A7   00000004    8        68\t00\t97\tCC\t00\t16\t39\tAA\r\n      2882  1FFFFFFF   00000004    8        00\t00\tFF\tFF\tFF\tFF\tFF\tFF\r\n      2872  1FFFFFFF   00000004    8        00\t00\tFF\tFF\tFF\tFF\tFF\tFF\r\n      2863  0CF102A7   00000004    8        30\t75\tE0\t2E\t80\tFF\tFF\tFD\r\n      2922  1FFFFFFF   00000004    8        00\t20\tFF\tFF\tFF\tFF\tFF\tFF\r\n      2912  1FFFFFFF   00000004    8        00\t20\tFF\tFF\tFF\tFF\tFF\tFF\r\n      2903  0CF102A7   00000004    8        30\t75\tE0\t2E\t80\tFF\tFF\tFD\r\n      2903  0CF101A7   00000004    8        68\t00\t97\tCC\t00\t16\t39\tAB\r\n      2902  1FFFFFFF   00000004    8        00\t20\tFF\tFF\tFF\tFF\tFF\tFF\r\n      2893  18F106A7   00000004    8        00\tF7\tFF\tFF\tFF\tFF\tFF\tAA\r\n      2892  1FFFFFFF   00000004    8        00\t20\tFF\tFF\tFF\tFF\tFF\tFF\r\n      2883  0CF102A7   00000004    8        30\t75\tE0\t2E\t80\tFF\tFF\tFD\r\n      2883  0CF101A7   00000004    8        68\t00\t97\tCC\t00\t16\t39\tAA\r\n      2882  1FFFFFFF   00000004    8        00\t00\tFF\tFF\tFF\tFF\tFF\tFF\r\n      2872  1FFFFFFF   00000004    8        00\t00\tFF\tFF\tFF\tFF\tFF\tFF\r\n      2923  0CF101A7   00000004    8        68\t00\t97\tCC\t00\t16\t39\tAC\r\n      2922  1FFFFFFF   00000004    8        00\t20\tFF\tFF\tFF\tFF\tFF\tFF\r\n      2912  1FFFFFFF   00000004    8        00\t20\tFF\tFF\tFF\tFF\tFF\tFF\r\n      2903  0CF102A7   00000004    8        30\t75\tE0\t2E\t80\tFF\tFF\tFD\r\n      2903  0CF101A7   00000004    8        68\t00\t97\tCC\t00\t16\t39\tAB\r\n      2902  1FFFFFFF   00000004    8        00\t20\tFF\tFF\tFF\tFF\tFF\tFF\r\n      2893  18F106A7   00000004    8        00\tF7\tFF\tFF\tFF\tFF\tFF\tAA\r\n      2892  1FFFFFFF   00000004    8        00\t20\tFF\tFF\tFF\tFF\tFF\tFF\r\n      2883  0CF102A7   00000004    8        30\t75\tE0\t2E\t80\tFF\tFF\tFD\r\n      2883  0CF101A7   00000004    8        68\t00\t97\tCC\t00\t16\t39\tAA\r\n      2882  1FFFFFFF   00000004    8        00\t00\tFF\tFF\tFF\tFF\tFF\tFF\r\n      2923  0CF102A7   00000004    8        30\t75\tE0\t2E\t80\tFF\tFF\tFD\r\n      2923  0CF101A7   00000004    8        68\t00\t97\tCC\t00\t16\t39\tAC\r\n      2922  1FFFFFFF   00000004    8        00\t20\tFF\tFF\tFF\tFF\tFF\tFF\r\n      2912  1FFFFFFF   00000004    8        00\t20\tFF\tFF\tFF\tFF\tFF\tFF\r\n      2903  0CF102A7   00000004    8        30\t75\tE0\t2E\t80\tFF\tFF\tFD\r\n      2903  0CF101A7   00000004    8        68\t00\t97\tCC\t00\t16\t39\tAB\r\n      2902  1FFFFFFF   00000004    8        00\t20\tFF\tFF\tFF\tFF\tFF\tFF\r\n      2893  18F106A7   00000004    8        00\tF7\tFF\tFF\tFF\tFF\tFF\tAA\r\n      2892  1FFFFFFF   00000004    8        00\t20\tFF\tFF\tFF\tFF\tFF\tFF\r\n      2883  0CF102A7   00000004    8        30\t75\tE0\t2E\t80\tFF\tFF\tFD\r\n      2883  0CF101A7   00000004    8        68\t00\t97\tCC\t00\t16\t39\tAA\r\n      2932  1FFFFFFF   00000004    8        00\t00\tFF\tFF\tFF\tFF\tFF\tFF\r\n      2923  0CF102A7   00000004    8        30\t75\tE0\t2E\t80\tFF\tFF\tFD\r\n      2923  0CF101A7   00000004    8        68\t00\t97\tCC\t00\t16\t39\tAC\r\n      2922  1FFFFFFF   00000004    8        00\t20\tFF\tFF\tFF\tFF\tFF\tFF\r\n      2912  1FFFFFFF   00000004    8        00\t20\tFF\tFF\tFF\tFF\tFF\tFF\r\n      2903  0CF102A7   00000004    8        30\t75\tE0\t2E\t80\tFF\tFF\tFD\r\n      2903  0CF101A7   00000004    8        68\t00\t97\tCC\t00\t16\t39\tAB\r\n      2902  1FFFFFFF   00000004    8        00\t20\tFF\tFF\tFF\tFF\tFF\tFF\r\n      2893  18F106A7   00000004    8        00\tF7\tFF\tFF\tFF\tFF\tFF\tAA\r\n      2892  1FFFFFFF   00000004    8        00\t20\tFF\tFF\tFF\tFF\tFF\tFF\r\n      2883  0CF102A7   00000004    8        30\t75\tE0\t2E\t80\tFF\tFF\tFD\r\n      2941  18F11FF0   00000004    8        FF\t3F\t90\t68\t88\t1B\t10\t5C\r\n      2932  1FFFFFFF   00000004    8        00\t00\tFF\tFF\tFF\tFF\tFF\tFF\r\n      2923  0CF102A7   00000004    8        30\t75\tE0\t2E\t80\tFF\tFF\tFD\r\n      2923  0CF101A7   00000004    8        68\t00\t97\tCC\t00\t16\t39\tAC\r\n      2922  1FFFFFFF   00000004    8        00\t20\tFF\tFF\tFF\tFF\tFF\tFF\r\n      2912  1FFFFFFF   00000004    8        00\t20\tFF\tFF\tFF\tFF\tFF\tFF\r\n      2903  0CF102A7   00000004    8        30\t75\tE0\t2E\t80\tFF\tFF\tFD\r\n      2903  0CF101A7   00000004    8        68\t00\t97\tCC\t00\t16\t39\tAB\r\n      2902  1FFFFFFF   00000004    8        00\t20\tFF\tFF\tFF\tFF\tFF\tFF\r\n      2893  18F106A7   00000004    8        00\tF7\tFF\tFF\tFF\tFF\tFF\tAA\r\n      2892  1FFFFFFF   00000004    8        00\t20\tFF\tFF\tFF\tFF\tFF\tFF\r\n      2942  18F120F0   00000004    8        2B\t75\t60\tB1\tB0\t01\tFF\tFF\r\n      2941  18F11FF0   00000004    8        FF\t3F\t90\t68\t88\t1B\t10\t5C\r\n      2932  1FFFFFFF   00000004    8        00\t00\tFF\tFF\tFF\tFF\tFF\tFF\r\n      2923  0CF102A7   00000004    8        30\t75\tE0\t2E\t80\tFF\tFF\tFD\r\n      2923  0CF101A7   00000004    8        68\t00\t97\tCC\t00\t16\t39\tAC\r\n      2922  1FFFFFFF   00000004    8        00\t20\tFF\tFF\tFF\tFF\tFF\tFF\r\n      2912  1FFFFFFF   00000004    8        00\t20\tFF\tFF\tFF\tFF\tFF\tFF\r\n      2903  0CF102A7   00000004    8        30\t75\tE0\t2E\t80\tFF\tFF\tFD\r\n      2903  0CF101A7   00000004    8        68\t00\t97\tCC\t00\t16\t39\tAB\r\n      2902  1FFFFFFF   00000004    8        00\t20\tFF\tFF\tFF\tFF\tFF\tFF\r\n      2893  18F106A7   00000004    8        00\tF7\tFF\tFF\tFF\tFF\tFF\tAA\r\n      2943  0CF101A7   00000004    8        68\t00\t97\tCC\t00\t16\t39\tAD\r\n      2942  18F120F0   00000004    8        2B\t75\t60\tB1\tB0\t01\tFF\tFF\r\n      2941  18F11FF0   00000004    8        FF\t3F\t90\t68\t88\t1B\t10\t5C\r\n      2932  1FFFFFFF   00000004    8        00\t00\tFF\tFF\tFF\tFF\tFF\tFF\r\n      2923  0CF102A7   00000004    8        30\t75\tE0\t2E\t80\tFF\tFF\tFD\r\n      2923  0CF101A7   00000004    8        68\t00\t97\tCC\t00\t16\t39\tAC\r\n      2922  1FFFFFFF   00000004    8        00\t20\tFF\tFF\tFF\tFF\tFF\tFF\r\n      2912  1FFFFFFF   00000004    8        00\t20\tFF\tFF\tFF\tFF\tFF\tFF\r\n      2903  0CF102A7   00000004    8        30\t75\tE0\t2E\t80\tFF\tFF\tFD\r\n      2903  0CF101A7   00000004    8        68\t00\t97\tCC\t00\t16\t39\tAB\r\n      2902  1FFFFFFF   00000004    8        00\t20\tFF\tFF\tFF\tFF\tFF\tFF\r\n      2943  0C3C4D4A   00000004    8        BE\tFF\tFF\t7F\t18\tFF\tFF\t55\r\n      2943  0CF101A7   00000004    8        68\t00\t97\tCC\t00\t16\t39\tAD\r\n      2942  18F120F0   00000004    8        2B\t75\t60\tB1\tB0\t01\tFF\tFF\r\n      2941  18F11FF0   00000004    8        FF\t3F\t90\t68\t88\t1B\t10\t5C\r\n      2932  1FFFFFFF   00000004    8        00\t00\tFF\tFF\tFF\tFF\tFF\tFF\r\n      2923  0CF102A7   00000004    8        30\t75\tE0\t2E\t80\tFF\tFF\tFD\r\n      2923  0CF101A7   00000004    8        68\t00\t97\tCC\t00\t16\t39\tAC\r\n      2922  1FFFFFFF   00000004    8        00\t20\tFF\tFF\tFF\tFF\tFF\tFF\r\n      2912  1FFFFFFF   00000004    8        00\t20\tFF\tFF\tFF\tFF\tFF\tFF\r\n      2903  0CF102A7   00000004    8        30\t75\tE0\t2E\t80\tFF\tFF\tFD\r\n      2903  0CF101A7   00000004    8        68\t00\t97\tCC\t00\t16\t39\tAB\r\n      2944  0CF102A7   00000004    8        30\t75\tE0\t2E\t80\tFF\tFF\tFD\r\n      2943  0C3C4D4A   00000004    8        BE\tFF\tFF\t7F\t18\tFF\tFF\t55\r\n      2943  0CF101A7   00000004    8        68\t00\t97\tCC\t00\t16\t39\tAD\r\n      2942  18F120F0   00000004    8        2B\t75\t60\tB1\tB0\t01\tFF\tFF\r\n      2941  18F11FF0   00000004    8        FF\t3F\t90\t68\t88\t1B\t10\t5C\r\n      2932  1FFFFFFF   00000004    8        00\t00\tFF\tFF\tFF\tFF\tFF\tFF\r\n      2923  0CF102A7   00000004    8        30\t75\tE0\t2E\t80\tFF\tFF\tFD\r\n      2923  0CF101A7   00000004    8        68\t00\t97\tCC\t00\t16\t39\tAC\r\n      2922  1FFFFFFF   00000004    8        00\t20\tFF\tFF\tFF\tFF\tFF\tFF\r\n      2912  1FFFFFFF   00000004    8        00\t20\tFF\tFF\tFF\tFF\tFF\tFF\r\n      2903  0CF102A7   00000004    8        30\t75\tE0\t2E\t80\tFF\tFF\tFD\r\n      2944  0CF103A7   00000004    8        17\t1F\t08\t60\tB1\t1F\t08\t55\r\n      2944  0CF102A7   00000004    8        30\t75\tE0\t2E\t80\tFF\tFF\tFD\r\n      2943  0C3C4D4A   00000004    8        BE\tFF\tFF\t7F\t18\tFF\tFF\t55\r\n      2943  0CF101A7   00000004    8        68\t00\t97\tCC\t00\t16\t39\tAD\r\n      2942  18F120F0   00000004    8        2B\t75\t60\tB1\tB0\t01\tFF\tFF\r\n      2941  18F11FF0   00000004    8        FF\t3F\t90\t68\t88\t1B\t10\t5C\r\n      2932  1FFFFFFF   00000004    8        00\t00\tFF\tFF\tFF\tFF\tFF\tFF\r\n      2923  0CF102A7   00000004    8        30\t75\tE0\t2E\t80\tFF\tFF\tFD\r\n      2923  0CF101A7   00000004    8        68\t00\t97\tCC\t00\t16\t39\tAC\r\n      2922  1FFFFFFF   00000004    8        00\t20\tFF\tFF\tFF\tFF\tFF\tFF\r\n      2912  1FFFFFFF   00000004    8        00\t20\tFF\tFF\tFF\tFF\tFF\tFF\r\n      2945  0CF104A7   00000004    8        F0\t60\t22\tFC\tFF\tFF\tFF\t55\r\n      2944  0CF103A7   00000004    
